vi "New Result From Call.vi"(8 "error in (no error)":errorcluster, 9 "input":i32, 10 "function":string, 11 "id":string) -> (0 "error out":errorcluster, 3 "result":refnum<class "result_from_call.lvclass">)   [LabVIEW 2015, in "result_from_call.lvclass"]
uses:
  result_from_call.lvclass
  result_from_call.lvclass/result_from_call.ctl
  result.lvclass
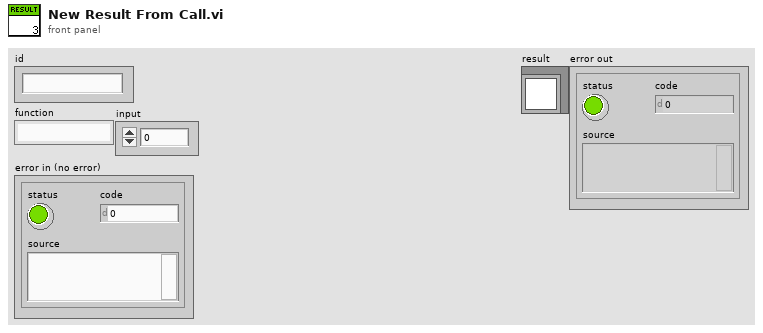
[diagram p1: front panel]
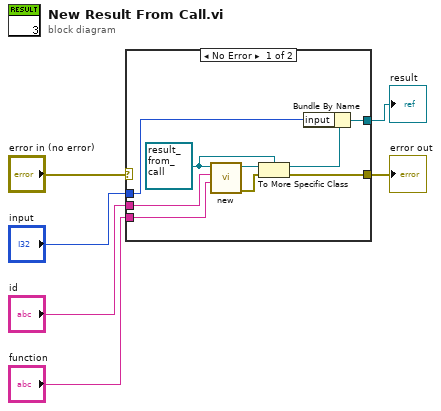
[diagram p0: block diagram]
diagram:
  n1 = case shown="No Error" "error in (no error)" {
    selector: "error in (no error)" -> [_ w16]
    tunnel: "function" -> [w15 _]
    tunnel: "id" -> [w14 _]
    tunnel: "input" -> [w9 _]
    tunnel: [w8 _] -> w3
    tunnel: [w7 w16] -> w1
    frame No Error {
      w12 = refnum<class "result_from_call.lvclass"> refnum ("result_from_call.lvclass")
      n2 = call "new.vi"("function"=w15, "id"=w14, "result"=w12) -> ("error Out"=w11:errorcluster, "result"=w13:refnum<class "result.lvclass">)  [unwired: 7 in]
      n3 = To More Specific Class(target class=w12, reference=w13, error in=w11) -> (specific class reference=w10:refnum<class "result_from_call.lvclass">, error out=w7:errorcluster)
      n4 = Bundle By Name(cluster=w10, "input"=w9) -> (w8:refnum<class "result_from_call.lvclass">)
    }
    frame Error {
    }
  }
  "result" <- w3
  "error out" <- w1
